vi "session_set_one_property_int32.vi"(6 "Skip setting if in Options string (F)":bool, 7 "Session Parameter Integer":T1=enum."Bin Data Chunk Size", 8 "error in":errorcluster caption="error in (no error)", 10 "Int32 value in":i32, 11 "VISA resource name":refnum<visa-resource-name>) -> (0 "error out":errorcluster, 2 "Set in the Options string":bool, 3 "VISA resource name out":refnum<visa-resource-name>)   [LabVIEW 2020, in "Rohde&Schwarz RTx Oscilloscopes.lvlib" / "rsidr_core.lvlib"]
doc: "OPC Timeout and VISA Timeout is not set if the 'int32 value in' is 0 or negative"
uses:
  rsidr_core.lvlib
  type_Session_Parameter_int32.ctl
  type_Error_Codes.ctl
  type_OPC_Wait_Mode.ctl
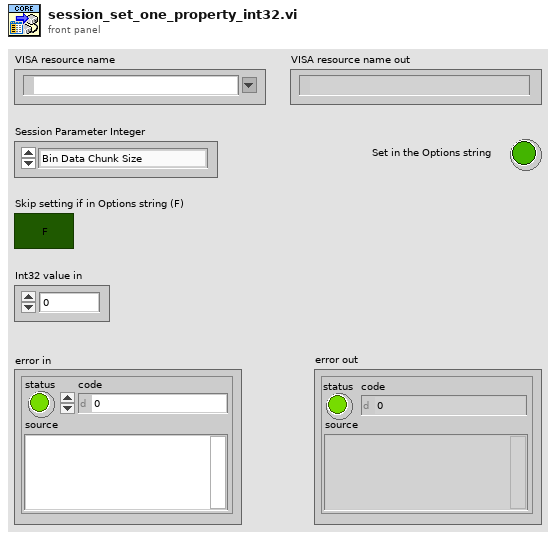
[diagram p1: front panel]
types:
  T1 = typedef "Rohde&Schwarz RTx Oscilloscopes.lvlib/rsidr_core.lvlib/type_Session_Parameter_int32.ctl" = enum16{"OPC Timeout", "Additional Flags", "Wait Before Write", "Wait Before Read", "Bin Data Chunk Size", "VISA Access Mode", "VISA Timeout", "Bin Float Number Format", "Bin Integer Number Format", "STBpollVISAtimeout", "OPCwaitMode"}
  T2 = typedef "Rohde&Schwarz RTx Oscilloscopes.lvlib/rsidr_core.lvlib/type_Session_Data.ctl" = cluster{"IDN string":string, "Instrument FW":string, "Instr type":string, "Instr type for err. msg.":string, "Installed Options":string[], "Ignore Error Messages":string, "Logging params":variant, "OPC Timeout":i32, "VISA Timeout":i32, "STB Poll VISA Timeout":i32, "Additional Flags":i32, "Wait Before Read":i32, "Wait Before Write":i32, "Option String Flags":i32, "IO Segment Size":i64, "VISA Access Mode":T3, "Interface Type":T4, "OPC Wait Mode":T5, "Bin Float Number  Format":T6, "Bin Integer Number Format":T7, "Simulate":bool, "VXIcapable":bool, "Duplicate Session":bool, "Add LF to Write":bool, "Logging":bool, "Fast Sweep":bool, "Query Instrument Status":bool, "Check Range":bool, "Check Options":bool, "OPC-sync Attr Writes":bool, "OPC-sync Attr Queries":bool}
  T3 = typedef "Rohde&Schwarz RTx Oscilloscopes.lvlib/rsidr_core.lvlib/type_VisaAccessMode.ctl" = u16
  T4 = typedef "Rohde&Schwarz RTx Oscilloscopes.lvlib/rsidr_core.lvlib/type_InterfaceType.ctl" = enum16{"Unknown", "GPIB", "VXI", "GPIB_VXI", "ASRL", "PXI", "TCPIP", "USB", "SOCKET"}
  T5 = typedef "Rohde&Schwarz RTx Oscilloscopes.lvlib/rsidr_core.lvlib/type_OPC_Wait_Mode.ctl" = enum16{"STBpolling", "STBpollingSlow", "STBpollingSuperSlow", "ServiceRequest", "OPCquery"}
  T6 = typedef "Rohde&Schwarz RTx Oscilloscopes.lvlib/rsidr_core.lvlib/type_Binary_Float_Number_Format.ctl" = enum16{"Float_4_Bytes_Swapped", "Float_4_Bytes", "Double_8_Bytes_Swapped", "Double_8_Bytes"}
  T7 = typedef "Rohde&Schwarz RTx Oscilloscopes.lvlib/rsidr_core.lvlib/type_Binary_Integer_Number_Format.ctl" = enum16{"Int32_4_Bytes_Swapped", "Int32_4 Bytes", "Int16_2_Bytes_Swapped", "Int16_2_Bytes"}
  T8 = typedef "Rohde&Schwarz RTx Oscilloscopes.lvlib/rsidr_core.lvlib/type_Error_Codes.ctl" = enum16{"No_error", "VISA_err_ResourceNotFound", "VISA_err_Timeout", "VISA_warn_MoreDataAvailable", "RS_err_MissingCallback", "RS_err_InvalidAttribute", "RS_err_InvalidValue", "RS_err_UnknownResource", "RS_err_AlreadyInitialized", "RS_err_InstrumentStatus", "RS_err_BadRepCapName", "RS_err_TypesMismatch", "RS_err_ValueNotSupported", "RS_err_InvalidRngTable", "RS_err_IDqueryFail", "RS_err_UnexpResponse", "VISA_warn_ConfigNotLoaded", "RS_err_AttributeNotReadable", "RS_err_AttributeNotWritable", "RS_err_InstrumentType", "RS_err_InstrumentOption", "VISA_err_InvalidSize", "RS_err_ReliabilityIndicator", "VISA_warn_UnknownStatus", "VISA_warn_TermCharRead", "VISA_err_IO_error", "RS_err_FunctionNotSupported", "VISA_warn_QueueEmpty"}
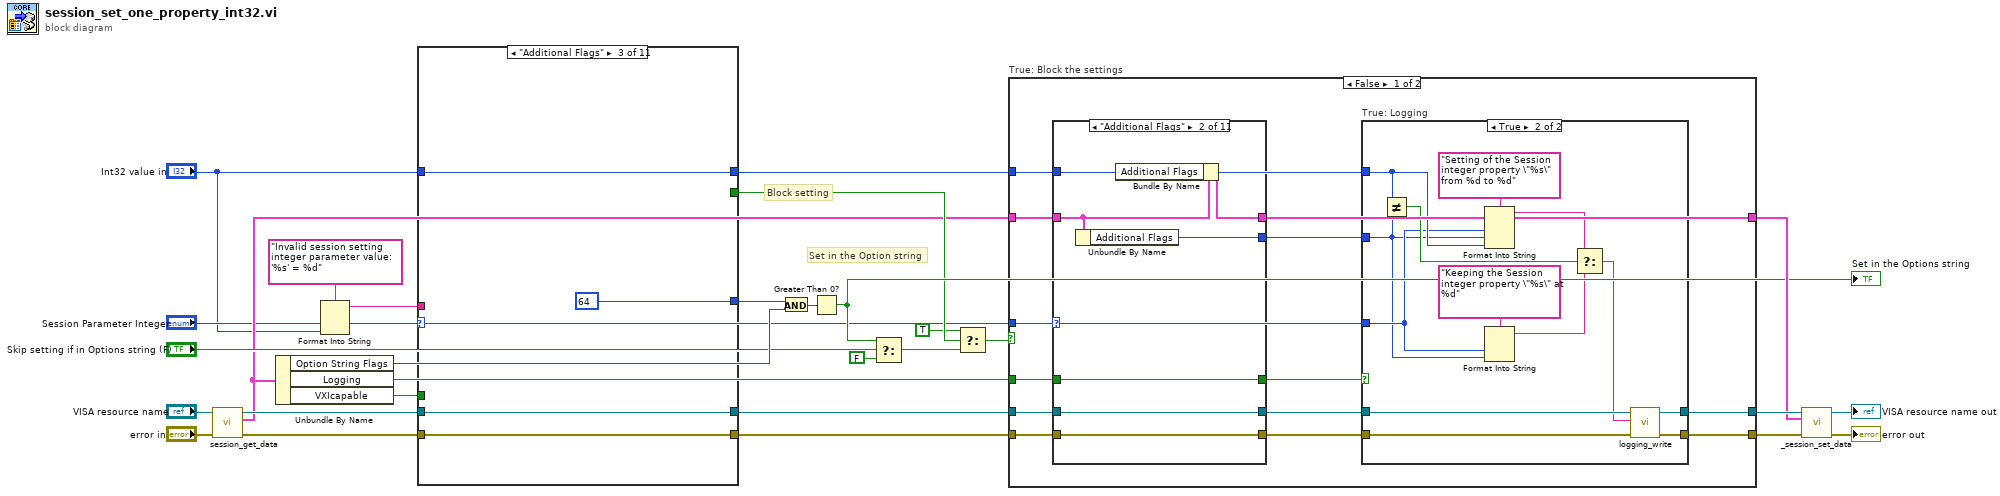
[diagram p0: block diagram]
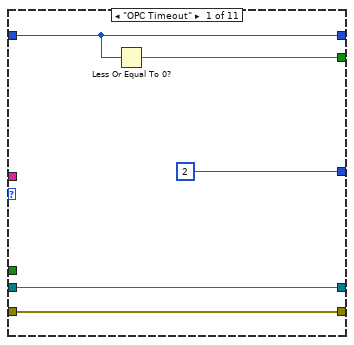
[diagram p2: hidden frame]
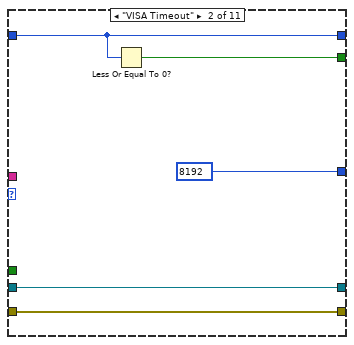
[diagram p3: hidden frame]
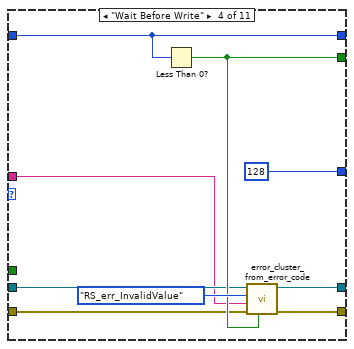
[diagram p4: hidden frame]
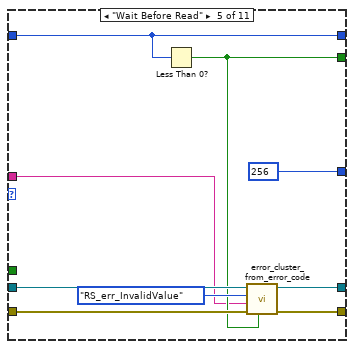
[diagram p5: hidden frame]
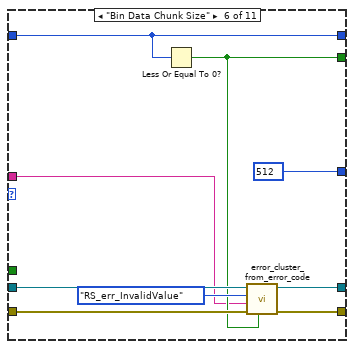
[diagram p6: hidden frame]
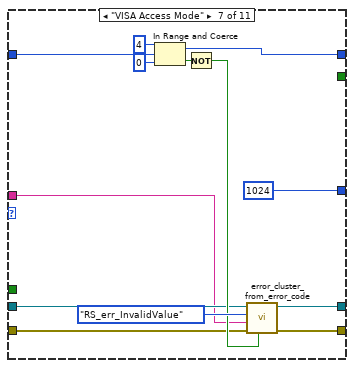
[diagram p7: hidden frame]
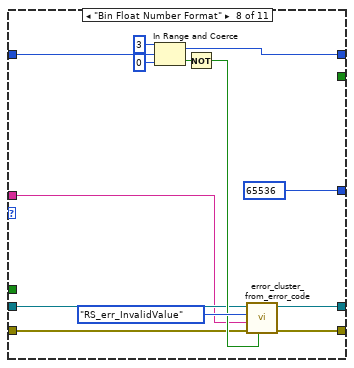
[diagram p8: hidden frame]
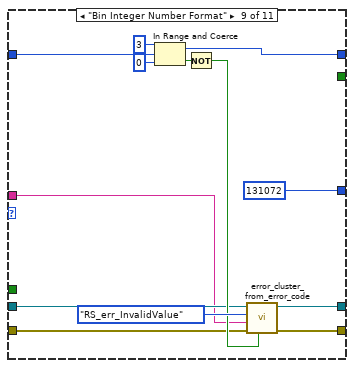
[diagram p9: hidden frame]
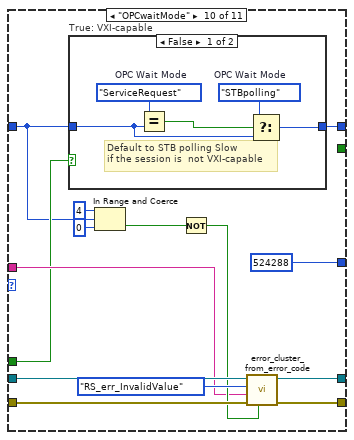
[diagram p10: hidden frame]
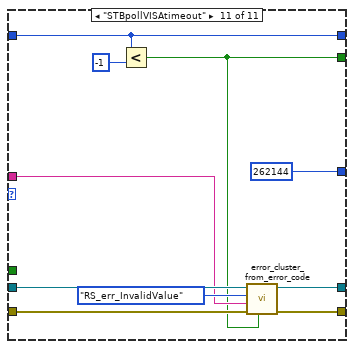
[diagram p12: hidden frame]
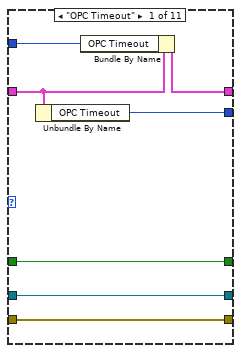
[diagram p14: hidden frame]
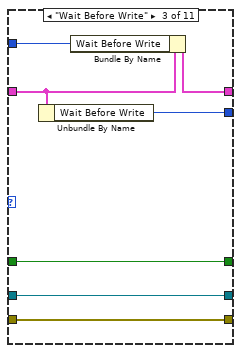
[diagram p15: hidden frame]
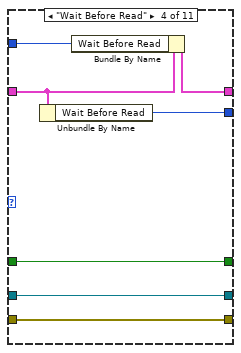
[diagram p16: hidden frame]
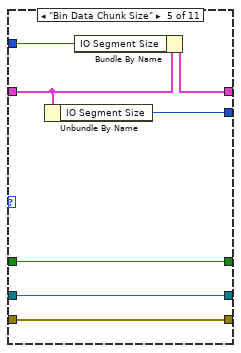
[diagram p17: hidden frame]
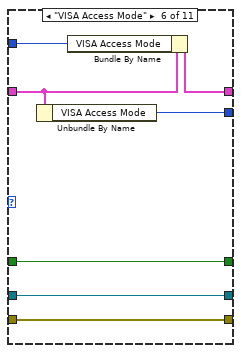
[diagram p18: hidden frame]
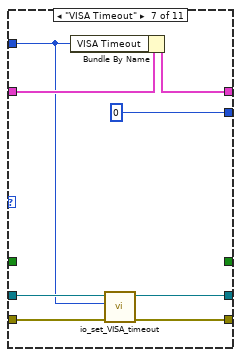
[diagram p19: hidden frame]
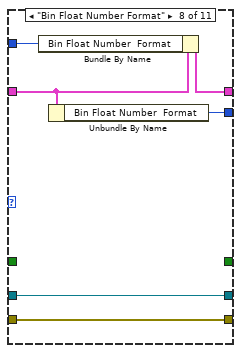
[diagram p20: hidden frame]
diagram:
  # "Block setting"
  # "Set in the Option string"
  n1 = call "session_get_data.vi"("error in"="error in", "VISA resource name"="VISA resource name") -> ("error out"=w9:errorcluster, "Session User Data out"=w6:T2, "VISA resource name out"=w10:refnum<visa-resource-name>)  [unwired: 6 in, 1 out]
  n2 = Unbundle By Name(w6) -> ("Option String Flags"=w20:i32, "Logging"=w19:bool, "VXIcapable"=w5:bool)
  n3 = Format Into String(format string="Invalid session setting integer parameter value: '%s' = %d", "Session Parameter Integer", "Int32 value in") -> (resulting string=w1:string)  [unwired: 2 in, 1 out]
  n4 = case shown="\"Additional Flags\"" "Session Parameter Integer" {
    tunnel: [2 8192 64 128 256 512 1024 65536 131072 524288 262144] -> w21
    tunnel: "Int32 value in" -> [w32 w35 w40 w51 w54 w63 w81 w94 w107 w113 w132]
    tunnel: [w33 w38 _ w49 w55 w64 _ _ _ _ w130] -> w14
    tunnel: [w32 w35 w40 w51 w54 w63 w74 w87 w100 w112 w132] -> w11
    tunnel: w10 -> [w30 w36 w41 w47 w58 w65 w77 w90 w103 w121 w137]
    tunnel: w9 -> [w31 w37 w42 w48 w59 w66 w78 w91 w104 w122 w138]
    tunnel: [w31 w37 w42 w46 w57 w67 w76 w89 w102 w120 w136] -> w8
    tunnel: [w30 w36 w41 w45 w56 w68 w75 w88 w101 w119 w135] -> w7
    tunnel: w5 -> [_ _ _ _ _ _ _ _ _ w114 _]
    tunnel: w1 -> [_ _ _ w44 w53 w62 w73 w86 w98 w115 w133]
    frame "OPC Timeout" {
      n5 = Less Or Equal To 0?(x=w32) -> (x <= 0?=w33:bool)
    }
    frame "VISA Timeout" {
      n6 = Less Or Equal To 0?(x=w35) -> (x <= 0?=w38:bool)
    }
    frame "Additional Flags" {
    }
    frame "Wait Before Write" {
      n7 = Less Than 0?(x=w51) -> (x < 0?=w49:bool)
      n8 = call "error_cluster_from_error_code.vi"("Error Creation Enabled (True)"=w49, "error in"=w48, "Error Message (\"\")"=w44, "Error Enum in"=type_Error_Codes."RS_err_InvalidValue", "VISA resource name"=w47) -> ("error out"=w46:errorcluster, "VISA resource name out"=w45:refnum<visa-resource-name>)  [unwired: 5 in]
    }
    frame "Wait Before Read" {
      n9 = Less Than 0?(x=w54) -> (x < 0?=w55:bool)
      n10 = call "error_cluster_from_error_code.vi"("Error Creation Enabled (True)"=w55, "error in"=w59, "Error Message (\"\")"=w53, "Error Enum in"=type_Error_Codes."RS_err_InvalidValue", "VISA resource name"=w58) -> ("error out"=w57:errorcluster, "VISA resource name out"=w56:refnum<visa-resource-name>)  [unwired: 5 in]
    }
    frame "Bin Data Chunk Size" {
      n11 = Less Or Equal To 0?(x=w63) -> (x <= 0?=w64:bool)
      n12 = call "error_cluster_from_error_code.vi"("Error Creation Enabled (True)"=w64, "error in"=w66, "Error Message (\"\")"=w62, "Error Enum in"=type_Error_Codes."RS_err_InvalidValue", "VISA resource name"=w65) -> ("error out"=w67:errorcluster, "VISA resource name out"=w68:refnum<visa-resource-name>)  [unwired: 5 in]
    }
    frame "VISA Access Mode" {
      n13 = In Range and Coerce(upper limit=4, x=w81, lower limit=0) -> (coerced(x)=w74:i32, In Range?=w80:bool)
      n14 = Not(x=w80) -> (.not. x?=w79:bool)
      n15 = call "error_cluster_from_error_code.vi"("Error Creation Enabled (True)"=w79, "error in"=w78, "Error Message (\"\")"=w73, "Error Enum in"=type_Error_Codes."RS_err_InvalidValue", "VISA resource name"=w77) -> ("error out"=w76:errorcluster, "VISA resource name out"=w75:refnum<visa-resource-name>)  [unwired: 5 in]
    }
    frame "Bin Float Number Format" {
      n16 = In Range and Coerce(upper limit=3, x=w94, lower limit=0) -> (coerced(x)=w87:i32, In Range?=w93:bool)
      n17 = Not(x=w93) -> (.not. x?=w92:bool)
      n18 = call "error_cluster_from_error_code.vi"("Error Creation Enabled (True)"=w92, "error in"=w91, "Error Message (\"\")"=w86, "Error Enum in"=type_Error_Codes."RS_err_InvalidValue", "VISA resource name"=w90) -> ("error out"=w89:errorcluster, "VISA resource name out"=w88:refnum<visa-resource-name>)  [unwired: 5 in]
    }
    frame "Bin Integer Number Format" {
      n19 = In Range and Coerce(upper limit=3, x=w107, lower limit=0) -> (coerced(x)=w100:i32, In Range?=w106:bool)
      n20 = Not(x=w106) -> (.not. x?=w105:bool)
      n21 = call "error_cluster_from_error_code.vi"("Error Creation Enabled (True)"=w105, "error in"=w104, "Error Message (\"\")"=w98, "Error Enum in"=type_Error_Codes."RS_err_InvalidValue", "VISA resource name"=w103) -> ("error out"=w102:errorcluster, "VISA resource name out"=w101:refnum<visa-resource-name>)  [unwired: 5 in]
    }
    frame "OPCwaitMode" {
      n22 = case "True: VXI-capable" shown="False" w114 {
        tunnel: w113 -> [w124 w129]
        tunnel: [w126 w129] -> w112
        frame False {
          w125 = type_OPC_Wait_Mode."STBpolling"  # OPC Wait Mode
          w128 = type_OPC_Wait_Mode."ServiceRequest"  # OPC Wait Mode
          # "Default to STB polling Slow\nif the session is  not VXI-capable"
          n23 = Equal?(x=w128, y=w124) -> (x = y?=w127:bool)
          n24 = Select(t=w125, s=w127, f=w124) -> (s? t:f=w126:i32)
        }
        frame True {
        }
      }
      n25 = In Range and Coerce(upper limit=4, x=w113, lower limit=0) -> (In Range?=w116:bool)  [unwired: 1 out]
      n26 = Not(x=w116) -> (.not. x?=w117:bool)
      n27 = call "error_cluster_from_error_code.vi"("Error Creation Enabled (True)"=w117, "error in"=w122, "Error Message (\"\")"=w115, "Error Enum in"=type_Error_Codes."RS_err_InvalidValue", "VISA resource name"=w121) -> ("error out"=w120:errorcluster, "VISA resource name out"=w119:refnum<visa-resource-name>)  [unwired: 5 in]
    }
    frame "STBpollVISAtimeout" {
      n28 = Less?(x=w132, y=-1) -> (x < y?=w130:bool)
      n29 = call "error_cluster_from_error_code.vi"("Error Creation Enabled (True)"=w130, "error in"=w138, "Error Message (\"\")"=w133, "Error Enum in"=type_Error_Codes."RS_err_InvalidValue", "VISA resource name"=w137) -> ("error out"=w136:errorcluster, "VISA resource name out"=w135:refnum<visa-resource-name>)  [unwired: 5 in]
    }
  }
  n30 = And(x=w21, y=w20) -> (x .and. y?=w29:i32)
  n31 = Greater Than 0?(x=w29) -> (x > 0?=w17:bool)
  "Set in the Options string" <- w17
  n32 = Select(t=w17, s="Skip setting if in Options string (F)", f=FALSE) -> (s? t:f=w13:bool)
  n33 = Select(t=TRUE, s=w14, f=w13) -> (s? t:f=w15:bool)
  n34 = case "True: Block the settings" shown="False" w15 {
    tunnel: "Session Parameter Integer" -> [w140 w244]
    tunnel: w6 -> [w152 w243]
    tunnel: w11 -> [w144 w245]
    tunnel: [w151 w243] -> w22
    tunnel: w8 -> [w150 w249]
    tunnel: w7 -> [w149 w248]
    tunnel: [w146 w247] -> w26
    tunnel: [w145 w246] -> w25
    tunnel: w19 -> [w143 w250]
    frame False {
      n35 = case shown="\"Additional Flags\"" w140 {
        tunnel: w144 -> [w174 w180 w187 w194 w201 w208 w211 w222 w228 w234 w240]
        tunnel: w152 -> [w169 w176 w183 w190 w197 w204 w213 w221 w227 w233 w239]
        tunnel: [w173 w181 w188 w195 w202 w209 w212 w223 w229 w235 w241] -> w151
        tunnel: w150 -> [w171 w179 w186 w193 w200 w207 w217 w218 w224 w230 w236]
        tunnel: w149 -> [w172 w178 w185 w192 w199 w206 w216 w219 w225 w231 w237]
        tunnel: [w171 w179 w186 w193 w200 w207 w215 w218 w224 w230 w236] -> w148
        tunnel: [w172 w178 w185 w192 w199 w206 w214 w219 w225 w231 w237] -> w147
        tunnel: w143 -> [w170 w177 w184 w191 w198 w205 _ _ _ _ _]
        tunnel: [w170 w177 w184 w191 w198 w205 _ _ _ _ _] -> w142
        tunnel: [w168 w175 w182 w189 w196 w203 i64 0 ("Bin Data Chunk Size") w220 w226 w232 w238] -> w141
        frame "OPC Timeout" {
          n36 = Unbundle By Name(w169) -> ("OPC Timeout"=w168:i32)
          n37 = Bundle By Name(cluster=w169, "OPC Timeout"=w174) -> (w173:T2)
        }
        frame "Additional Flags" {
          n38 = Unbundle By Name(w176) -> ("Additional Flags"=w175:i32)
          n39 = Bundle By Name(cluster=w176, "Additional Flags"=w180) -> (w181:T2)
        }
        frame "Wait Before Write" {
          n40 = Unbundle By Name(w183) -> ("Wait Before Write"=w182:i32)
          n41 = Bundle By Name(cluster=w183, "Wait Before Write"=w187) -> (w188:T2)
        }
        frame "Wait Before Read" {
          n42 = Unbundle By Name(w190) -> ("Wait Before Read"=w189:i32)
          n43 = Bundle By Name(cluster=w190, "Wait Before Read"=w194) -> (w195:T2)
        }
        frame "Bin Data Chunk Size" {
          n44 = Unbundle By Name(w197) -> ("IO Segment Size"=w196:i64)
          n45 = Bundle By Name(cluster=w197, "IO Segment Size"=w201) -> (w202:T2)
        }
        frame "VISA Access Mode" {
          n46 = Unbundle By Name(w204) -> ("VISA Access Mode"=w203:T3)
          n47 = Bundle By Name(cluster=w204, "VISA Access Mode"=w208) -> (w209:T2)
        }
        frame "VISA Timeout" {
          n48 = Bundle By Name(cluster=w213, "VISA Timeout"=w211) -> (w212:T2)
          n49 = call "io_set_VISA_timeout.vi"("error in"=w217, "VISA Timeout"=w211, "VISA resource name"=w216) -> ("error out"=w215:errorcluster, "VISA resource name out"=w214:refnum<visa-resource-name>)  [unwired: 6 in, 1 out]
        }
        frame "Bin Float Number Format" {
          n50 = Bundle By Name(cluster=w221, "Bin Float Number  Format"=w222) -> (w223:T2)
          n51 = Unbundle By Name(w221) -> ("Bin Float Number  Format"=w220:T6)
        }
        frame "Bin Integer Number Format" {
          n52 = Bundle By Name(cluster=w227, "Bin Integer Number Format"=w228) -> (w229:T2)
          n53 = Unbundle By Name(w227) -> ("Bin Integer Number Format"=w226:T7)
        }
        frame "STBpollVISAtimeout" {
          n54 = Bundle By Name(cluster=w233, "STB Poll VISA Timeout"=w234) -> (w235:T2)
          n55 = Unbundle By Name(w233) -> ("STB Poll VISA Timeout"=w232:i32)
        }
        frame "OPCwaitMode" {
          n56 = Bundle By Name(cluster=w239, "OPC Wait Mode"=w240) -> (w241:T2)
          n57 = Unbundle By Name(w239) -> ("OPC Wait Mode"=w238:T5)
        }
      }
      n58 = case "True: Logging" shown="True" w142 {
        tunnel: w141 -> [_ w155]
        tunnel: w144 -> [_ w157]
        tunnel: w140 -> [_ w156]
        tunnel: w148 -> [w153 w163]
        tunnel: w147 -> [w154 w162]
        tunnel: [w153 w161] -> w146
        tunnel: [w154 w160] -> w145
        frame False {
        }
        frame True {
          n59 = Not Equal?(x=w157, y=w155) -> (x != y?=w158:bool)
          n60 = Format Into String(format string="Setting of the Session integer property \"%s\" from %d to %d", w156, w155, w157) -> (resulting string=w166:string)  [unwired: 2 in, 1 out]
          n61 = Format Into String(format string="Keeping the Session integer property \"%s\" at %d", w156, w155) -> (resulting string=w167:string)  [unwired: 2 in, 1 out]
          n62 = Select(t=w166, s=w158, f=w167) -> (s? t:f=w159:string)
          n63 = call "logging_write.vi"("error in"=w163, "String to write"=w159, "VISA resource name"=w162) -> ("error out"=w161:errorcluster, "VISA resource name out"=w160:refnum<visa-resource-name>)  [unwired: 7 in]
        }
      }
    }
    frame True {
      n64 = case shown="\"OPCwaitMode\"" w244 {
        tunnel: w243 -> [w252 w254 w256 w258 w260 w262 w264 w266 w268 w270 w272]
        tunnel: [w251 w253 w255 w257 w259 w261 w263 w265 w267 w269 w271] -> w242
        frame "OPC Timeout" {
          n65 = Unbundle By Name(w252) -> ("OPC Timeout"=w251:i32)
        }
        frame "Additional Flags" {
          n66 = Unbundle By Name(w254) -> ("Additional Flags"=w253:i32)
        }
        frame "Wait Before Write" {
          n67 = Unbundle By Name(w256) -> ("Wait Before Write"=w255:i32)
        }
        frame "Wait Before Read" {
          n68 = Unbundle By Name(w258) -> ("Wait Before Read"=w257:i32)
        }
        frame "Bin Data Chunk Size" {
          n69 = Unbundle By Name(w260) -> ("IO Segment Size"=w259:i64)
        }
        frame "VISA Access Mode" {
          n70 = Unbundle By Name(w262) -> ("VISA Access Mode"=w261:T3)
        }
        frame "VISA Timeout" {
          n71 = Unbundle By Name(w264) -> ("VISA Timeout"=w263:i32)
        }
        frame "Bin Float Number Format" {
          n72 = Unbundle By Name(w266) -> ("Bin Float Number  Format"=w265:T6)
        }
        frame "Bin Integer Number Format" {
          n73 = Unbundle By Name(w268) -> ("Bin Integer Number Format"=w267:T7)
        }
        frame "STBpollVISAtimeout" {
          n74 = Unbundle By Name(w270) -> ("STB Poll VISA Timeout"=w269:i32)
        }
        frame "OPCwaitMode" {
          n75 = Unbundle By Name(w272) -> ("OPC Wait Mode"=w271:T5)
        }
      }
      n76 = case "True: Logging" shown="True" w250 {
        tunnel: w249 -> [w274 w279]
        tunnel: w248 -> [w273 w278]
        tunnel: [w274 w277] -> w247
        tunnel: [w273 w276] -> w246
        tunnel: w244 -> [_ w283]
        tunnel: w245 -> [_ w280]
        tunnel: w242 -> [_ w275]
        frame False {
        }
        frame True {
          n77 = Format Into String(format string="Setting of the Session integer property \"%s\" to value %d blocked, keeping the value %d", w283, w280, w275) -> (resulting string=w281:string)  [unwired: 2 in, 1 out]
          n78 = call "logging_write.vi"("error in"=w279, "String to write"=w281, "VISA resource name"=w278) -> ("error out"=w277:errorcluster, "VISA resource name out"=w276:refnum<visa-resource-name>)  [unwired: 7 in]
        }
      }
    }
  }
  n79 = call "_session_set_data.vi"("error in"=w26, "Session User Data in"=w22, "VISA resource name"=w25) -> ("error out"=→"error out":errorcluster, "VISA resource name out"=→"VISA resource name out":refnum<visa-resource-name>)  [unwired: 7 in]
